vi "Asylum_TipDown.vi"() -> ()   [LabVIEW 2016]
panel:
  in  "Z SetPoint":dbl
  in  "Application":refnum<k7>
  in  "error in (no error)":errorcluster
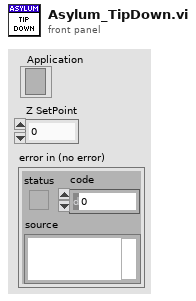
[diagram p1: front panel]
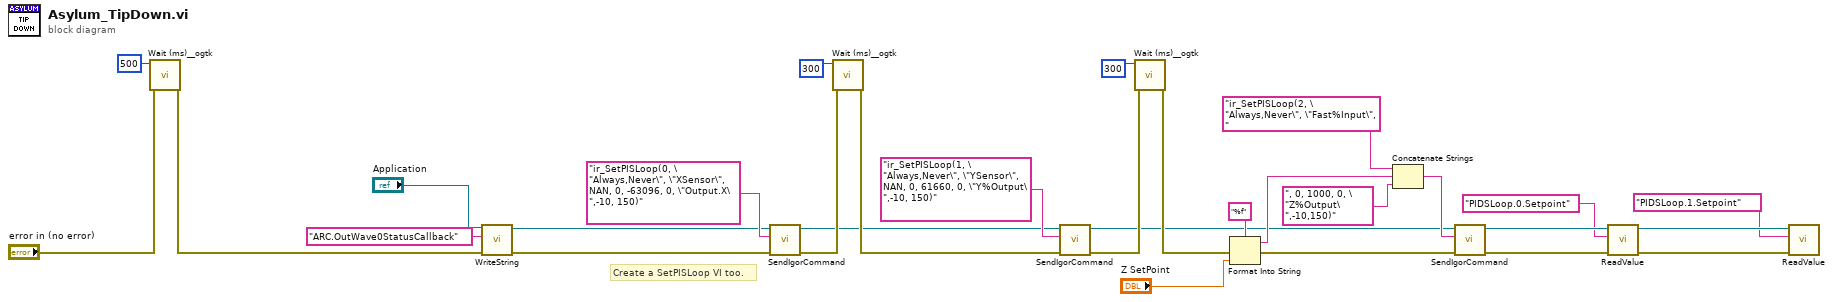
[diagram p0: block diagram]
diagram:
  # "Create a SetPISLoop VI too."
  n1 = call <userlib>:"Wait (ms)__ogtk.vi"("error in (no error)"="error in (no error)", "milliseconds to wait"=u32 500) -> ("error out"=w12:errorcluster)  [unwired: 8 in, 1 out]
  n2 = call "WriteString.vi"("error in (no error)"=w12, "StringToWrite"="ARC.OutWave0StatusCallback", "Application"="Application") -> ("error out"=w11:errorcluster, "Application"=w8:refnum<k7>)  [unwired: 7 in]
  n3 = call "SendIgorCommand.vi"("error in (no error)"=w11, "command"="ir_SetPISLoop(0, \"Always,Never\", \"XSensor\", NAN, 0, -63096, 0, \"Output.X\",-10, 150)", "Application"=w8) -> ("error out"=w26:errorcluster, "Application"=w23:refnum<k7>)  [unwired: 5 in, 2 out]
  n4 = call <userlib>:"Wait (ms)__ogtk.vi"("error in (no error)"=w26, "milliseconds to wait"=u32 300) -> ("error out"=w25:errorcluster)  [unwired: 8 in, 1 out]
  n5 = call "SendIgorCommand.vi"("error in (no error)"=w25, "command"="ir_SetPISLoop(1, \"Always,Never\", \"YSensor\", NAN, 0, 61660, 0, \"Y%Output\",-10, 150)", "Application"=w23) -> ("error out"=w18:errorcluster, "Application"=w13:refnum<k7>)  [unwired: 5 in, 2 out]
  n6 = call <userlib>:"Wait (ms)__ogtk.vi"("error in (no error)"=w18, "milliseconds to wait"=u32 300) -> ("error out"=w17:errorcluster)  [unwired: 8 in, 1 out]
  n7 = Format Into String(format string="%f", error in=w17, "Z SetPoint") -> (resulting string=w16:string, error out=w15:errorcluster)  [unwired: 1 in]
  n8 = Concatenate Strings("ir_SetPISLoop(2, \"Always,Never\", \"Fast%Input\", " ("string"), w16, ", 0, 1000, 0, \"Z%Output\",-10,150)" ("string")) -> (w14:string)
  n9 = call "SendIgorCommand.vi"("error in (no error)"=w15, "command"=w14, "Application"=w13) -> ("error out"=w7:errorcluster, "Application"=w6:refnum<k7>)  [unwired: 5 in, 2 out]
  n10 = call "ReadValue.vi"("error in (no error)"=w7, "Value"="PIDSLoop.0.Setpoint" ("command"), "Application"=w6) -> ("error out"=w2:errorcluster, "Application"=w4:refnum<k7>)  [unwired: 6 in, 1 out]
  n11 = call "ReadValue.vi"("error in (no error)"=w2, "Value"="PIDSLoop.1.Setpoint" ("command"), "Application"=w4) -> ()  [unwired: 6 in, 3 out]
